vi "goToPointA.vi"(5 "Fora do circulo":bool, 6 "Raio":dbl=123.0, 7 "Target":dbl[](array[numeric]), 8 "error in (no error)":errorcluster, 9 "Game":refnum<class "Game.lvclass">, 10 "Robot in":refnum<class "Robot.lvclass">, 11 "KickToSkill in":refnum<class "KickToSkill.lvclass">) -> (0 "error out":errorcluster, 2 "Robot out":refnum<class "Robot.lvclass">, 3 "KickToSkill out":refnum<class "KickToSkill.lvclass">)   [LabVIEW 2023, in "KickToSkill.lvclass"]
uses:
  KickToSkill.lvclass
  Robot_class/Robot.lvclass
  C:/Users/ebert/Desktop/roboime/SSL_AI/Object_class/Object.lvclass
  Game_class/Game.lvclass
  Game_class/Game.lvclass/Game.ctl
  Object_class/Object.lvclass/Object.ctl
  Robot_class/Robot.lvclass/Robot.ctl
  <vilib>/Analysis/coordinate.llb/2D Cartesian Coordinate Shift (Scalar).vi
  <vilib>/Analysis/coordinate.llb/2D Cartesian Coordinate Rotation (Scalar).vi
  Object_class/Read x.vi
  Object_class/Read y.vi
  Robot_class/Write dest_x.vi
  Robot_class/Write dest_y.vi
  Robot_class/Write dest_orientation.vi
  Game_class/Read NewParameters.vi
  Object_class/Read position(x,y).vi
  Game_class/Read BallRef.vi
  Ball_class/Ball.lvclass
  <vilib>/Analysis/NI_AALPro.lvlib
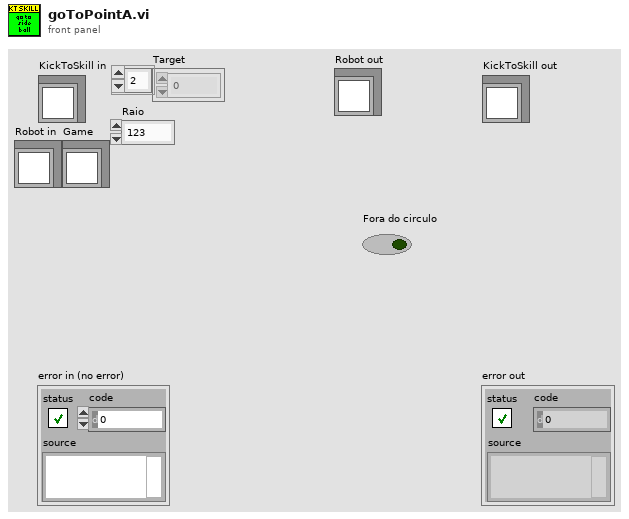
[diagram p1: front panel]
types:
  T1 = typedef "NewParameters.ctl" = cluster{"PenaltyDistance":dbl, "DistanceAttackerToBackBall":dbl, "Division":enum16{"Div B", "Div A"}, "DistanceToAvoidyEnemyRobot":dbl, "BallPlacementDistance":dbl, "DisatanceBehindBallToStealBall":dbl, "MaxDistanceToPositionKickoff":dbl, "BlockEnemyTarget":bool, "MaxStopVAng":dbl, "DistanceMarkerToEnemy":dbl, "IgnoreDribblerContact":bool, "DistanceToBeginEnemyPosession":dbl, "GoToBallWhenEnemyNotMoving":bool, "EnemyDistanceToReduceVelocity":dbl, "TurnOnEnemyDistanceToReduceVelocity":bool, "EnemyDistanceToShootOutBall":dbl, "DefenseKickBall":bool, "MoreKickToGoal? (0-0.3)":dbl, "ChipKickInEnemyField":bool, "ShootOutRobotId":dbl, "FieldLenghtDenominatorInShootOut":dbl, "AdjustPositionInBallPlacement":bool, "PowerGodPass":dbl, "VelocityAbortEnemyPos":dbl, "MaxDistToBeginPass":dbl, "MinDistToBeginPass":dbl, "VelocityInDirects":dbl, "BadDribblerIDs":i32[], "NewKickToDistanceAroundBall":dbl, "PowerAvoidColisionMarker":dbl, "DistanceToAvoidColisionMarker":dbl, "AvoidBallKick":dbl, "DistanceTryKick":dbl, "SuicideKickDIstance":dbl, "AdjustFirstKickDistance":dbl, "AvoidAimLessKick":dbl, "DistanceToAvoidyEnemyShootRobot ":dbl, "NumberOfMarkers":dbl, "PotField":bool, "PIDLateral":bool, "MinDistanceFirstKickX":dbl, "MinDistanceFirstKickY":dbl, "FractionOfDistToTouchGround\nAfterChipKick":dbl, "FractionOfKickxWhen\nComposedWithKickz":dbl, "Style":T2, "MoveInTurnState":bool, "DistFromEnemyToConsider\nMoveInTurnState":dbl, "CascadePID":bool, "TurnAroundParameters":cluster{"Radius":dbl, "Multiplier":dbl, "ChordAngle":dbl}, "SafeDriveVel":dbl, "DistanceToGoToBackBall":dbl, "minDistanceToNotFinish\nEnemyPossession":dbl, "OneTouchShot":cluster{"angleFactor":dbl, "maxAngle":dbl, "Attack":bool, "Defense":bool}, "OpenAngleToGoal":cluster{"minAngle":dbl, "maxAngle":dbl, "minEvaluation":dbl}, "ShotInterception":cluster{"shotSpeed":dbl, "minEnemySpeed":dbl, "maxEnemySpeed":dbl, "minEvaluation":dbl}, "AllyTeamArray":T3[], "maxDefendersNumber":i32, "Zone":cluster{"GuardPositionArray":dbl[][], "ZoneMidField":dbl[], "CenterForwardWidth":dbl}, "MinEvaluationToShoot":dbl, "PassInterception":cluster{"maxPassSpeed":dbl, "minPassSpeed":dbl, "minEnemySpeed":dbl, "chipPassDistance":dbl, "chipPassEvaluation":dbl, "minEvaluation":dbl, "maxEnemySpeed":dbl}, "PassDistance":cluster{"maxDistance":dbl, "minDistance":dbl}, "receiverSpeed":dbl, "maxBallSpeed":dbl, "slackTime":dbl, "Turning radius":dbl, "Turning v_ang":dbl, "AlignError":cluster{"Distance":dbl, "Orientation":dbl, "V_norm(m/s)":dbl, "V_ang (rad/s)":dbl}, "RobotRadius":dbl, "KickerDistance":dbl, "keeper angle  to cover goalpost":dbl}
  T2 = typedef "Style.ctl" = enum16{"Insanity", "Offensive", "Defensive"}
  T3 = typedef "AllyTeam.ctl" = enum16{"Keeper", "Defender", "Attacker"}
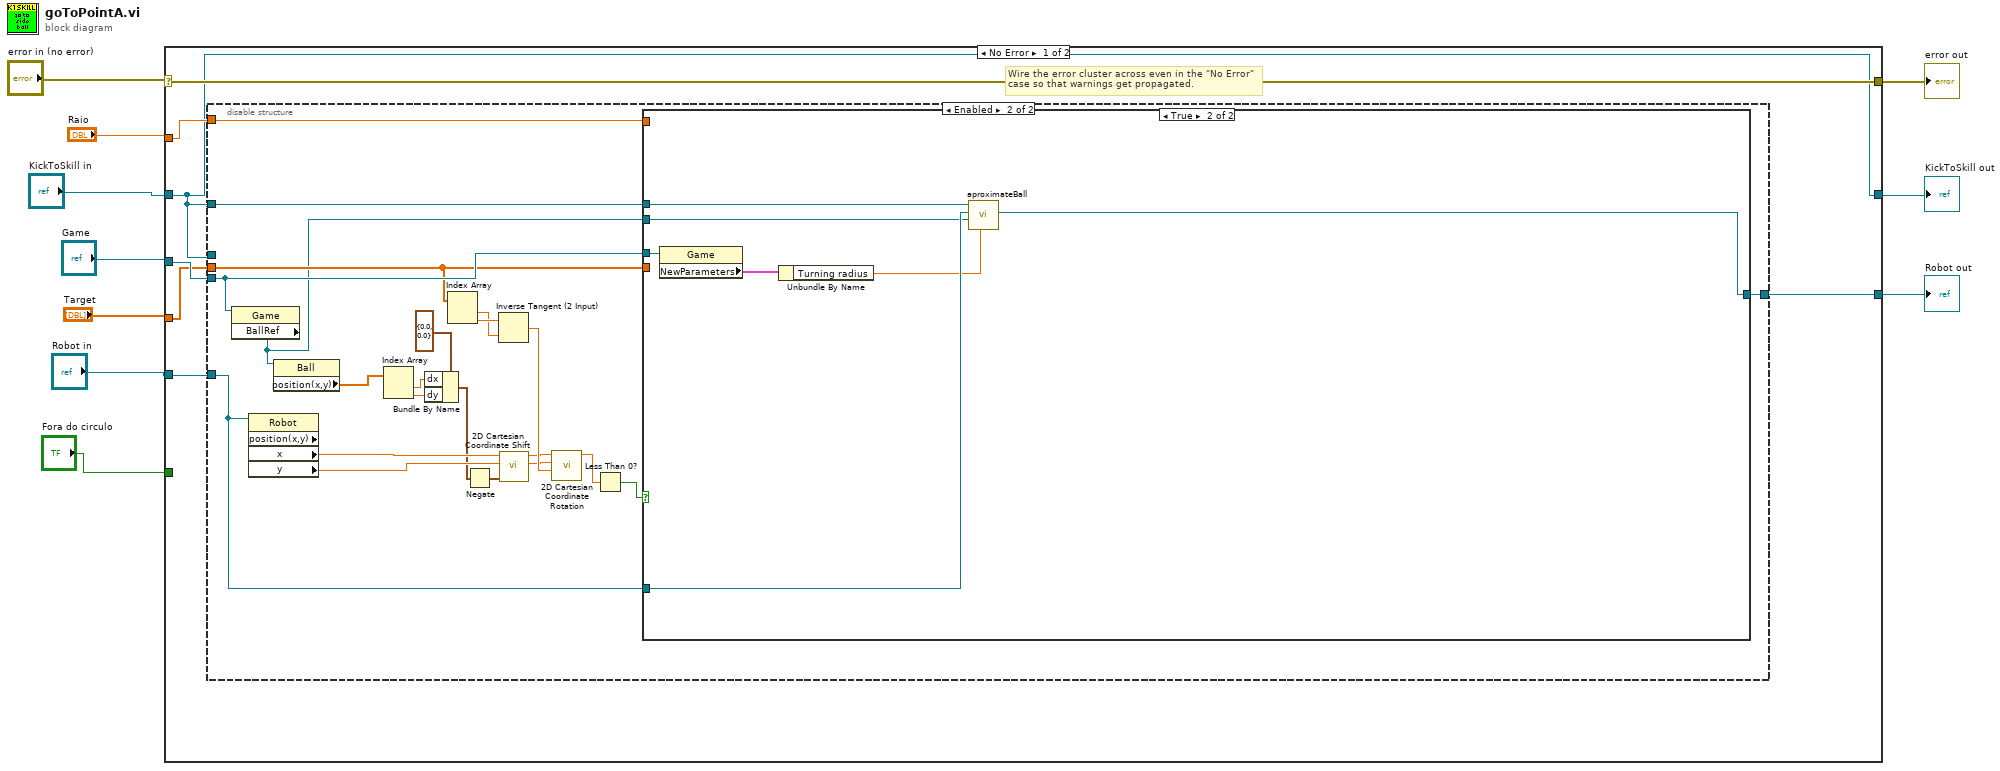
[diagram p0: block diagram]
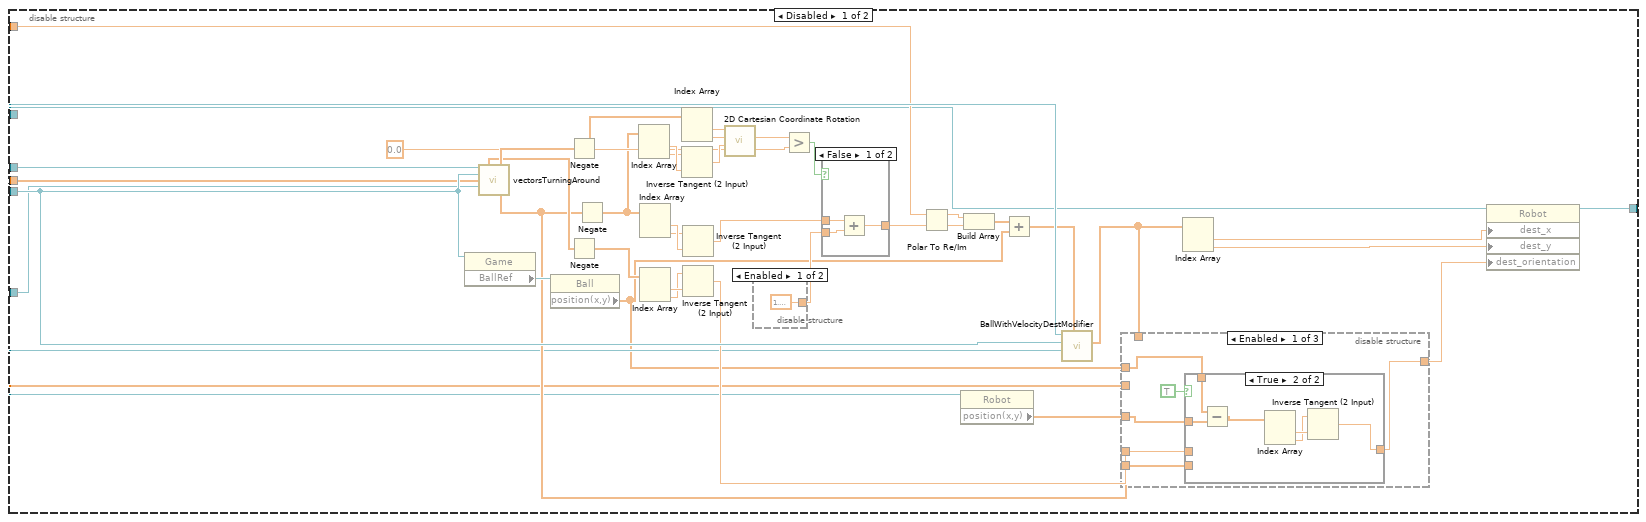
[diagram p2: hidden frame]
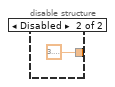
[diagram p3: hidden frame]
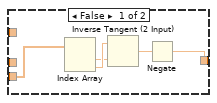
[diagram p4: hidden frame]
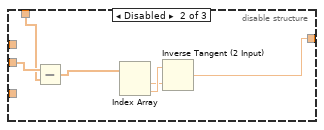
[diagram p5: hidden frame]
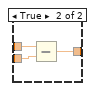
[diagram p7: hidden frame]
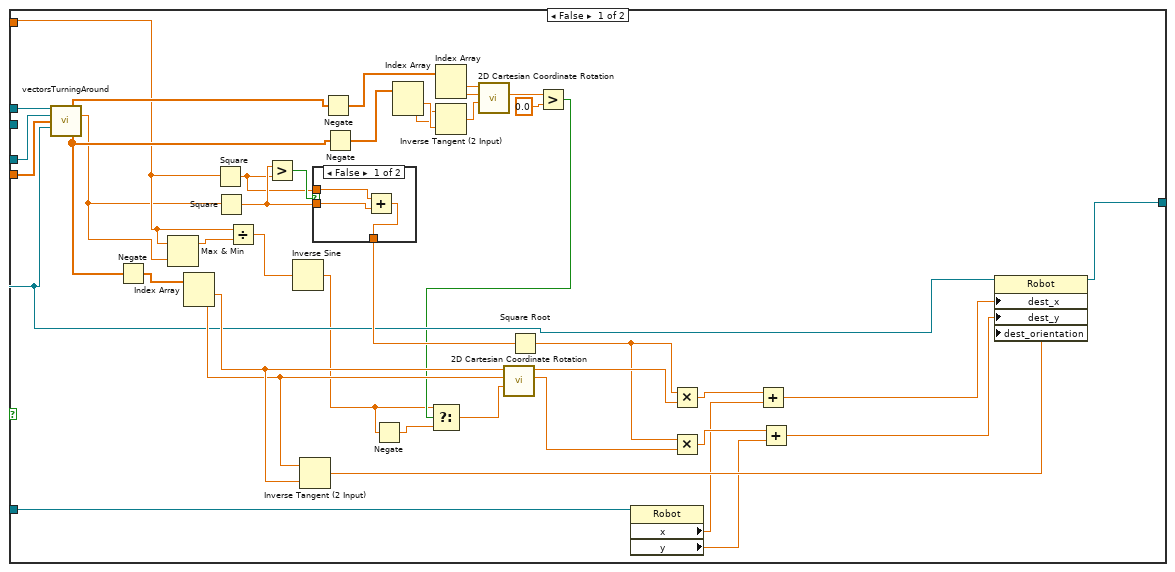
[diagram p8: hidden frame]
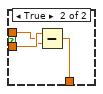
[diagram p9: hidden frame]
diagram:
  n1 = case shown="No Error" "error in (no error)" {
    selector: "error in (no error)" -> [w17 w166]
    tunnel: [w17 w166] -> w9
    tunnel: [w11 w165] -> w7
    tunnel: "KickToSkill in" -> [w11 w165]
    tunnel: "Game" -> [w15 _]
    tunnel: "Target" -> [w12 _]
    tunnel: "Robot in" -> [w13 w164]
    tunnel: [w16 w164] -> w3
    tunnel: "Raio" -> [w14 _]
    tunnel: "Fora do circulo" -> [_ _]
    frame No Error {
      # "Wire the error cluster across even in the \"No Error\"\ncase so that warnings get propagated."
      n2 = disable-structure shown="Enabled" {
        disable-tunnel: [w56 w108] -> w16
        disable-tunnel: w15 -> [w29 w105]
        disable-tunnel: w11 -> [w28 _]
        disable-tunnel: w14 -> [w23 w107]
        disable-tunnel: w13 -> [w22 w104]
        disable-tunnel: w12 -> [w19 w101]
        disable-tunnel: w11 -> [_ w109]
        frame Disabled {
          n3 = property class="Game"(reference=w29) -> ("BallRef"=w40:refnum<class "Ball.lvclass">)  [unwired: 1 in, 2 out]
          n4 = call "vectorsTurningAround.vi"("KickToSkill in"=w28, "Game"=w29, "Target"=w19, "Robot in"=w22) -> ("Robot - Target"=w33:dbl[], "Ball - Target"=w54:dbl[], "Robot - Ball"=w24:dbl[])  [unwired: 4 in, 5 out]
          n5 = property class="Ball"(reference=w40) -> ("position(x,y)"=w18:dbl[])  [unwired: 1 in, 2 out]
          n6 = Negate(x=w54) -> (-x=w53:dbl[])
          n7 = Negate(x=w33) -> (-x=w32:dbl[])
          n8 = Negate(x=w24) -> (-x=w43:dbl[])
          n9 = Index Array(array=w43) -> (element #1=w50:dbl, element #2=w49:dbl)  [unwired: 2 in]
          n10 = Index Array(array=w43) -> (element #1=w45:dbl, element #2=w44:dbl)  [unwired: 2 in]
          n11 = Index Array(array=w32) -> (element #1=w31:dbl, element #2=w30:dbl)  [unwired: 2 in]
          n12 = Index Array(array=w53) -> (element #1=w52:dbl, element #2=w51:dbl)  [unwired: 2 in]
          n13 = Inverse Tangent (2 Input)(1:w50, 2:w49) -> (0:w55:dbl)
          n14 = Inverse Tangent (2 Input)(1:w45, 2:w44) -> (0:w42:dbl)
          n15 = Inverse Tangent (2 Input)(1:w31, 2:w30) -> (0:w26:dbl)
          n16 = call-poly <vilib>:"2D Cartesian Coordinate Rotation.vi"("theta"=w55, "y"=w51, "x"=w52) -> ("y out"=w48:dbl)  [unwired: 6 in, 2 out]
          n17 = disable-structure shown="Enabled" {
            disable-tunnel: [1.5707963267948966 3.141592653589793] -> w41
            frame Enabled {
            }
            frame Disabled {
            }
          }
          n18 = Greater?(x=w48, y=0.0) -> (0:w46:bool)
          n19 = case shown="False" w46 {
            tunnel: w42 -> [w84 w87]
            tunnel: w41 -> [w83 w86]
            tunnel: [w82 w85] -> w37
            frame False {
              n20 = Add(x=w84, y=w83) -> (x+y=w82:dbl)
            }
            frame True {
              n21 = Subtract(x=w87, y=w86) -> (x-y=w85:dbl)
            }
          }
          n22 = Polar To Re/Im(2:w37, 3:w23) -> (0:w38:dbl, 1:w39:dbl)
          n23 = property class="Robot"(reference=w22) -> ("position(x,y)"=w20:dbl[])  [unwired: 1 in, 2 out]
          n24 = Build Array(w39, w38) -> (w34:dbl[])
          n25 = Add(x=w34, y=w18) -> (x+y=w27:dbl[])
          n26 = call "BallWithVelocityDestModifier.vi"("destino original"=w27, "Robot in"=w22, "Game"=w29, "KickToSkill in"=w28) -> ("destino com velocidade"=w21:dbl[])  [unwired: 5 in, 2 out]
          n27 = disable-structure shown="Enabled" {
            disable-tunnel: w26 -> [w64 _ _]
            disable-tunnel: [w63 w76 _] -> w25
            disable-tunnel: w24 -> [w62 _ _]
            disable-tunnel: w21 -> [_ w80 _]
            disable-tunnel: w20 -> [w61 _ _]
            disable-tunnel: w19 -> [_ w81 _]
            disable-tunnel: w18 -> [w59 _ _]
            frame Enabled {
              n28 = case shown="True" TRUE {
                tunnel: w64 -> [_ _]
                tunnel: [w65 w70] -> w63
                tunnel: w62 -> [w66 _]
                tunnel: w59 -> [_ w72]
                tunnel: w61 -> [_ w71]
                frame False {
                  n29 = Index Array(array=w66) -> (element #1=w68:dbl, element #2=w69:dbl)  [unwired: 2 in]
                  n30 = Inverse Tangent (2 Input)(1:w68, 2:w69) -> (0:w67:dbl)
                  n31 = Negate(x=w67) -> (-x=w65:dbl)
                }
                frame True {
                  n32 = Subtract(x=w72, y=w71) -> (x-y=w75:dbl[])
                  n33 = Index Array(array=w75) -> (element #1=w74:dbl, element #2=w73:dbl)  [unwired: 2 in]
                  n34 = Inverse Tangent (2 Input)(1:w74, 2:w73) -> (0:w70:dbl)
                }
              }
            }
            frame Disabled {
              n35 = Subtract(x=w81, y=w80) -> (x-y=w77:dbl[])
              n36 = Index Array(array=w77) -> (element #1=w78:dbl, element #2=w79:dbl)  [unwired: 2 in]
              n37 = Inverse Tangent (2 Input)(1:w78, 2:w79) -> (0:w76:dbl)
            }
            frame Disabled {
            }
          }
          n38 = Index Array(array=w21) -> (element #1=w36:dbl, element #2=w35:dbl)  [unwired: 2 in]
          n39 = property class="Robot"(reference=w22, "dest_x"=w36, "dest_y"=w35, "dest_orientation"=w25) -> (reference out=w56:refnum<class "Robot.lvclass">)  [unwired: 1 in, 1 out]
        }
        frame Enabled {
          n40 = property class="Game"(reference=w105) -> ("BallRef"=w93:refnum<class "Ball.lvclass">)  [unwired: 1 in, 2 out]
          n41 = property class="Robot" props=["position(x,y)", "x", "y"](reference=w104) -> ("x"=w103:dbl, "y"=w102:dbl)  [unwired: 1 in, 3 out]
          n42 = property class="Ball"(reference=w93) -> ("position(x,y)"=w92:dbl[])  [unwired: 1 in, 2 out]
          n43 = Index Array(array=w92) -> (element #1=w91:dbl, element #2=w90:dbl)  [unwired: 2 in]
          n44 = Bundle By Name(cluster=cluster{"dx":dbl, "dy":dbl} {"dx"=0.0, "dy"=0.0} ("shift"), "dx"=w91, "dy"=w90) -> (w89:cluster{"dx":dbl, "dy":dbl})
          n45 = Index Array(array=w101) -> (element #1=w99:dbl, element #2=w100:dbl)  [unwired: 2 in]
          n46 = Negate(x=w89) -> (-x=w88:cluster{"dx":dbl, "dy":dbl})
          n47 = Inverse Tangent (2 Input)(1:w99, 2:w100) -> (0:w98:dbl)
          n48 = call-poly <vilib>:"2D Cartesian Coordinate Shift.vi"("shift"=w88, "y"=w102, "x"=w103) -> ("y out"=w96:dbl, "x out"=w97:dbl)  [unwired: 6 in, 1 out]
          n49 = call-poly <vilib>:"2D Cartesian Coordinate Rotation.vi"("theta"=w98, "y"=w96, "x"=w97) -> ("x out"=w95:dbl)  [unwired: 6 in, 2 out]
          n50 = Less Than 0?(x=w95) -> (x < 0?=w94:bool)
          n51 = case shown="True" w94 {
            tunnel: w109 -> [w150 w162]
            tunnel: w101 -> [w149 _]
            tunnel: w105 -> [w148 w161]
            tunnel: [w134 w157] -> w108
            tunnel: w104 -> [w122 w163]
            tunnel: w107 -> [w115 _]
            tunnel: w93 -> [_ w158]
            frame False {
              n52 = call "vectorsTurningAround.vi"("KickToSkill in"=w150, "Game"=w148, "Target"=w149, "Robot in"=w122) -> ("Ball - Target"=w141:dbl[], "Robot - Ball norm"=w114:dbl, "Robot - Ball"=w136:dbl[])  [unwired: 4 in, 5 out]
              n53 = Negate(x=w136) -> (-x=w135:dbl[])
              n54 = Max & Min(x=w115, y=w114) -> (max(x,y)=w113:dbl)  [unwired: 1 out]
              n55 = Index Array(array=w135) -> (element #1=w130:dbl, element #2=w129:dbl)  [unwired: 2 in]
              n56 = Square(x=w115) -> (x^2=w110:dbl)
              n57 = Square(x=w114) -> (x^2=w111:dbl)
              n58 = Divide(x=w115, y=w113) -> (x/y=w137:dbl)
              n59 = Greater?(x=w111, y=w110) -> (0:w112:bool)
              n60 = Inverse Sine(1:w137) -> (0:w116:dbl)
              n61 = Inverse Tangent (2 Input)(1:w130, 2:w129) -> (0:w128:dbl)
              n62 = case shown="False" w112 {
                tunnel: [w151 w156] -> w127
                tunnel: w111 -> [w152 w155]
                tunnel: w110 -> [w153 w154]
                frame False {
                  n63 = Add(x=w153, y=w152) -> (x+y=w151:dbl)
                }
                frame True {
                  n64 = Subtract(x=w155, y=w154) -> (x-y=w156:dbl)
                }
              }
              n65 = Negate(x=w141) -> (-x=w146:dbl[])
              n66 = Negate(x=w136) -> (-x=w140:dbl[])
              n67 = Negate(x=w116) -> (-x=w117:dbl)
              n68 = Index Array(array=w140) -> (element #1=w139:dbl, element #2=w138:dbl)  [unwired: 2 in]
              n69 = Index Array(array=w146) -> (element #1=w145:dbl, element #2=w144:dbl)  [unwired: 2 in]
              n70 = Inverse Tangent (2 Input)(1:w139, 2:w138) -> (0:w147:dbl)
              n71 = call-poly <vilib>:"2D Cartesian Coordinate Rotation.vi"("theta"=w147, "y"=w144, "x"=w145) -> ("y out"=w143:dbl)  [unwired: 6 in, 2 out]
              n72 = Square Root(x=w127) -> (sqrt(x)=w132:dbl)
              n73 = Greater?(x=w143, y=0.0) -> (0:w118:bool)
              n74 = Select(t=w116, s=w118, f=w117) -> (s? t:f=w119:dbl)
              n75 = call-poly <vilib>:"2D Cartesian Coordinate Rotation.vi"("theta"=w119, "y"=w129, "x"=w130) -> ("y out"=w131:dbl, "x out"=w133:dbl)  [unwired: 6 in, 1 out]
              n76 = property class="Robot"(reference=w122) -> ("x"=w121:dbl, "y"=w120:dbl)  [unwired: 1 in, 2 out]
              n77 = Multiply(x=w132, y=w133) -> (x*y=w126:dbl)
              n78 = Multiply(x=w132, y=w131) -> (x*y=w125:dbl)
              n79 = Add(x=w126, y=w121) -> (x+y=w124:dbl)
              n80 = Add(x=w125, y=w120) -> (x+y=w123:dbl)
              n81 = property class="Robot"(reference=w122, "dest_x"=w124, "dest_y"=w123, "dest_orientation"=w128) -> (reference out=w134:refnum<class "Robot.lvclass">)  [unwired: 1 in, 1 out]
            }
            frame True {
              n82 = property class="Game"(reference=w161) -> ("NewParameters"=w160:T1)  [unwired: 1 in, 2 out]
              n83 = Unbundle By Name(w160) -> ("Turning radius"=w159:dbl)
              n84 = call "aproximateBall.vi"("Radius"=w159, "Ball"=w158, "Robot"=w163, "KickToSkill in"=w162) -> ("Robot out"=w157:refnum<class "Robot.lvclass">)  [unwired: 5 in, 2 out]
            }
          }
        }
      }
    }
    frame Error {
    }
  }
  "error out" <- w9
  "KickToSkill out" <- w7
  "Robot out" <- w3
